vi "G#Debugger_Start.vi"(0 "application reference":refnum<vi>, 5 "error in (no error)":errorcluster) -> (19 "error out":errorcluster)   [LabVIEW 2017, in "G#Debugger.lvlib"]
doc: "Starts the G# Debugger in the same application instance as this VI executes."
uses:
  <vilib>/addons/_AddQ/G#Debugger/G#Debugger.lvlib
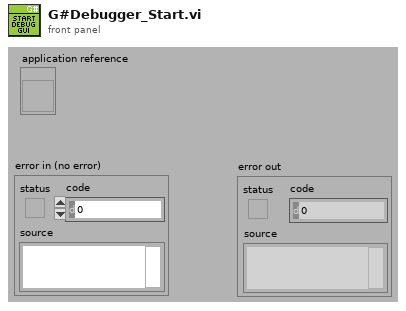
[diagram p1: front panel]
types:
  T1 = enum32{"Bad", "Idle", "Run top level", "Running"}
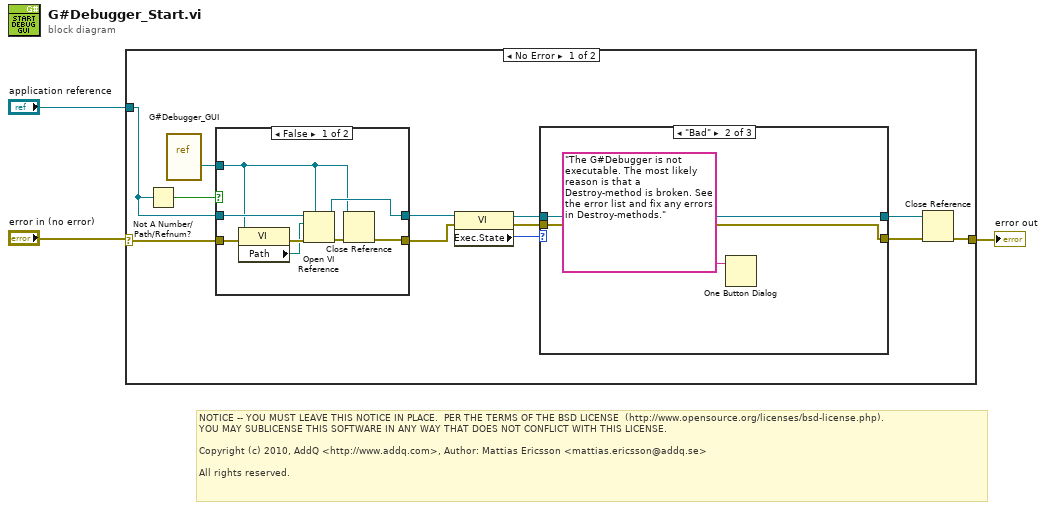
[diagram p0: block diagram]
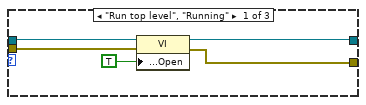
[diagram p3: hidden frame]
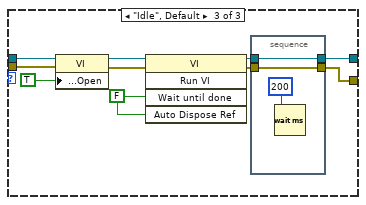
[diagram p4: hidden frame]
diagram:
  # "NOTICE -- YOU MUST LEAVE THIS NOTICE IN PLACE.  PER THE TERMS OF THE BSD LICENSE  (http://www.opensource.org/licenses/bsd-license.php).\nYOU MAY SUBLICENSE THIS SOFTWARE IN ANY WAY THAT DOES NOT CONFLICT WITH THIS LICENSE.\n\nCopyright (c) 2010, AddQ <http://www.addq.com>, Author: Mattias Ericsson <mattias.ericsson@addq.se>\n\nAll rights reserved."
  n1 = case shown="No Error" "error in (no error)" {
    selector: "error in (no error)" -> [w8 w47]
    tunnel: [w4 w47] -> w3
    tunnel: "application reference" -> [w5 _]
    frame No Error {
      n2 = Not A Number/Path/Refnum?(number/path/refnum=w5) -> (NaN/Path/Refnum?=w6:bool)
      n3 = vi-ref <vilib>:"G#Debugger_GUI.vi"() -> (w7:refnum<vi>)
      n4 = case shown="False" w6 {
        tunnel: [w20 w25] -> w14
        tunnel: [w23 w24] -> w13
        tunnel: w8 -> [w19 w25]
        tunnel: w7 -> [w17 w24]
        tunnel: w5 -> [w22 _]
        frame False {
          n5 = property class="VI"(reference=w17, error in=w19) -> (error out=w18:errorcluster, "Path"=w16:path)  [unwired: 1 out]
          n6 = Open VI Reference(type specifier VI Refnum (for type only)=w17, application reference (local)=w22, vi path=w16, error in (no error)=w18) -> (vi reference=w23:refnum<vi>, error out=w21:errorcluster)  [unwired: 2 out]
          n7 = Close Reference(reference=w17, error in (no error)=w21) -> (error out=w20:errorcluster)
        }
        frame True {
        }
      }
      n8 = property class="VI"(reference=w13, error in=w14) -> (reference out=w11:refnum<vi>, error out=w12:errorcluster, "Exec.State"=w10:T1)
      n9 = case shown="\"Bad\"" w10 {
        tunnel: [w26 w32 w43] -> w9
        tunnel: [w27 w33 w42] -> w15
        tunnel: w12 -> [w29 w32 w36]
        tunnel: w11 -> [w30 w33 w37]
        frame "Run top level", "Running" {
          n10 = property class="VI"(reference=w30, error in=w29, "Front Panel.Open"=TRUE ("Front Panel Window:Open")) -> (reference out=w27:refnum<vi>, error out=w26:errorcluster)
        }
        frame "Bad" {
          n11 = One Button Dialog(message="The G#Debugger is not executable. The most likely reason is that a Destroy-method is broken. See the error list and fix any errors in Destroy-methods.") -> ()  [unwired: 1 in, 1 out]
        }
        frame "Idle", Default {
          w39 = FALSE ("Wait Until Done")
          n12 = property class="VI"(reference=w37, error in=w36, "Front Panel.Open"=TRUE ("Front Panel Window:Open")) -> (reference out=w35:refnum<vi>, error out=w34:errorcluster)
          n13 = invoke class="VI" method="Run VI"(reference=w35, error in=w34, "Wait until done"=w39, "Auto Dispose Ref"=w39) -> (reference out=w41:refnum<vi>, error out=w40:errorcluster)  [unwired: 1 in, 3 out]
          n14 = stacked-sequence {
            tunnel: w40 -> [w45]
            tunnel: w41 -> [w46]
            tunnel: [w46] -> w42
            tunnel: [w45] -> w43
            frame #0 {
              n15 = Wait (ms)(milliseconds to wait=u32 200) -> ()  [unwired: 1 out]
            }
          }
        }
      }
      n16 = Close Reference(reference=w15, error in (no error)=w9) -> (error out=w4:errorcluster)
    }
    frame Error {
    }
  }
  "error out" <- w3
